vi "Enable Peak.vi"(8 "error in (no error)":errorcluster, 10 "Enable Peak Test (F: False)":bool, 11 "VISA resource name":refnum<visa-resource-name>) -> (0 "error out":errorcluster, 3 "VISA resource name out":refnum<visa-resource-name>)   [LabVIEW 2019, in "BK Precision 8500B Series.lvlib"]
doc: "Enables or disables the Peak Test Function."
uses:
  <instrlib>/BK Precision 8500B Series/BK Precision 8500B Series.lvlib
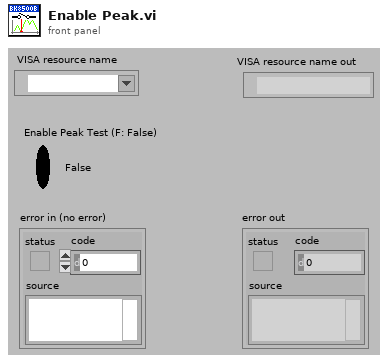
[diagram p1: front panel]
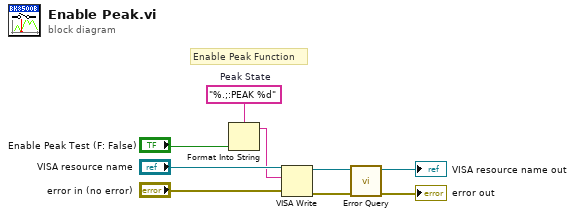
[diagram p0: block diagram]
diagram:
  w9 = "%.;:PEAK %d"  # Peak State
  # "Enable Peak Function"
  n1 = Format Into String(format string=w9, "Enable Peak Test (F: False)") -> (resulting string=w3:string)  [unwired: 2 in, 1 out]
  n2 = VISA Write(VISA resource name="VISA resource name", write buffer=w3, error in (no error)="error in (no error)") -> (VISA resource name out=w2:refnum<visa-resource-name>, error out=w1:errorcluster)  [unwired: 1 out]
  n3 = call <instrlib>:"Error Query.vi"("error in (no error)"=w1, "VISA resource name"=w2) -> ("error out"=→"error out":errorcluster, "VISA resource name out"=→"VISA resource name out":refnum<visa-resource-name>)  [unwired: 6 in, 2 out]
